vi "GetMenuItem.vi"(8 "error in (no error)":errorcluster, 10 "Tag":string, 11 "MenuMap":map{string, T2}(c390)) -> (0 "error out":errorcluster, 1 "Short Cut":T1, 2 "Item Tags":string[](array[string]), 3 "Item Names":string[](array[string]), 4 "Checked":bool, 5 "Picture":refnum<class "Image.lvclass">, 6 "Enable":bool, 7 "Hilite Picture":refnum<class "Image.lvclass">)   [LabVIEW 2021, in "Menu.lvlib" / "Menu.lvclass"]
uses:
  Menu.lvclass
  Menu.lvclass/Menu.ctl
  <vilib>/Utility/miscctls.llb/LVMenuShortCut.ctl
  MenuItems.ctl
  Picture2D/src/Picture/Image.lvclass
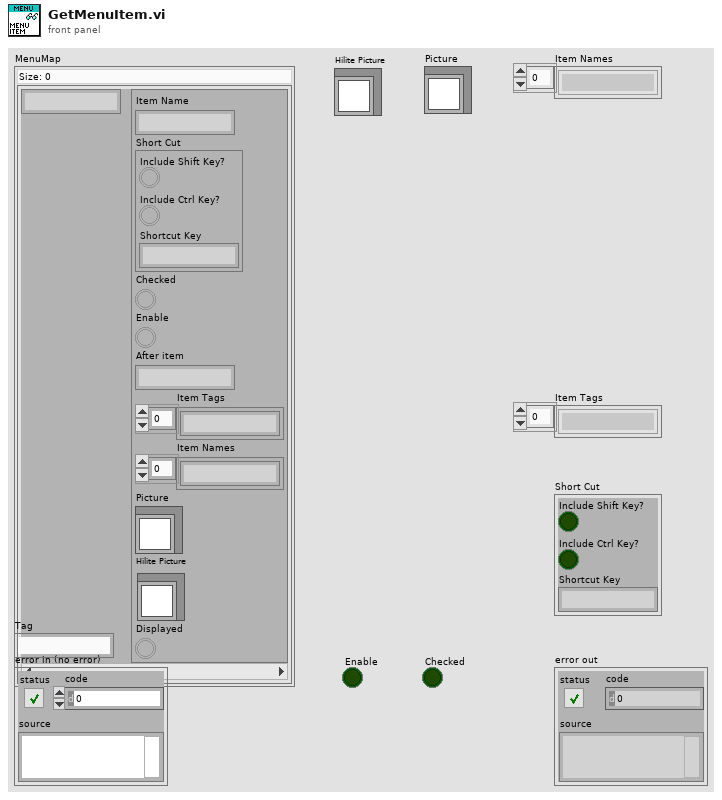
[diagram p1: front panel]
types:
  T1 = typedef "LVMenuShortCut.ctl" = cluster{"Include Shift Key?":bool, "Include Ctrl Key?":bool, "Shortcut Key":string}
  T2 = typedef "Menu.lvlib/Menu.lvclass/MenuItems.ctl" = cluster{"Item Name":string, "Short Cut":T1, "Checked":bool, "Enable":bool, "After item":string, "Item Tags":string[], "Item Names":string[], "Picture":refnum<class "Image.lvclass">, "Hilite Picture":refnum<class "Image.lvclass">, "Displayed":bool}
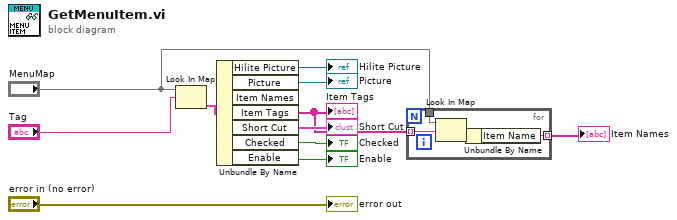
[diagram p0: block diagram]
diagram:
  n1 = Look In Map(map="MenuMap", key="Tag") -> (value=w11:T2)  [unwired: 1 in, 1 out]
  n2 = Unbundle By Name(w11) -> ("Hilite Picture"=→"Hilite Picture":refnum<class "Image.lvclass">, "Picture"=→"Picture":refnum<class "Image.lvclass">, "Item Tags"=w2:string[], "Short Cut"=→"Short Cut":T1, "Checked"=→"Checked":bool, "Enable"=→"Enable":bool)  [unwired: 1 out]
  "Item Tags" <- w2
  n3 = for {
    tunnel: "MenuMap" -> [w15]
    tunnel: w2 -> [w14] mode=indexing
    tunnel: [w12] -> w1 mode=indexing
    n4 = Look In Map(map=w15, key=w14) -> (value=w13:T2)  [unwired: 1 in, 1 out]
    n5 = Unbundle By Name(w13) -> ("Item Name"=w12:string)
  }
  "Item Names" <- w1
  "error out" <- "error in (no error)"
